vi "Maya2000 - set N coadd and integr time.vi"(4 "Intgration time\n[us]":u32=44444, 6 "numberOfScans\nToAverage":u32=1 min=1 step=1, 8 "error in (no error)":errorcluster, 9 "Array index of UV\nspectrometers":T1, 10 "Maya2000 basic values":T2[](array[typedef]), 11 ".NET Refnum in":refnum<k24>) -> (0 "error out":errorcluster, 1 "This instruments index":i32, 2 "This Maya´\nbasic info":T2, 3 ".NET Refnum out":refnum<k24>)   [LabVIEW 2015]
uses:
  Maya2000 Typedefs/Maya2000 basic info.ctl
  C:/Program Files (x86)/Ocean Optics/OmniDriver/OOI_HOME/NETOmniDriver-NET40.dll
  Maya2000 Typedefs/Basic info-array index of UV spectometers.ctl
  <vilib>/GPower/Error/Library/ErrorType.vi
  <vilib>/GPower/Error/Library/SplitAppended.vi
  <vilib>/GPower/Error/Library/SubVIs/ExplanationToError.vi
  <vilib>/dlg_ctls.llb/Space Constant.vi
  <vilib>/Utility/error.llb/Error Cluster From Error Code.vi
  <vilib>/Utility/error.llb/Trim Whitespace.vi
  <vilib>/Utility/error.llb/Error Code Database.vi
  <vilib>/GPower/Error/Library/SubVIs/SetStatus.vi
  <vilib>/GPower/Error/Library/AppendErrors.vi
  <vilib>/GPower/Error/Library/Append/AppendSingle.vi
  <vilib>/ErrorRing/Error Ring.xnode
  <vilib>/GPower/Error/GPError.lvlib
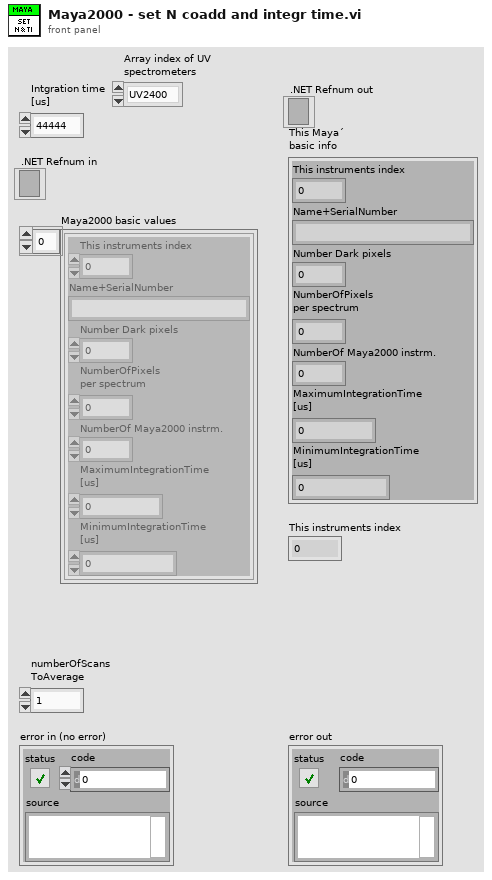
[diagram p1: front panel]
types:
  T1 = typedef "Basic info-array index of UV spectometers.ctl" = enum32{"UV2400", "UV600"}
  T2 = typedef "Maya2000 basic info.ctl" = cluster{"This instruments index":i32, "Name+SerialNumber":string, "Number Dark pixels":i32, "NumberOfPixels\nper spectrum":i32, "NumberOf Maya2000 instrm.":i32, "MaximumIntegrationTime\n[us]":i32, "MinimumIntegrationTime\n[us]":i32}
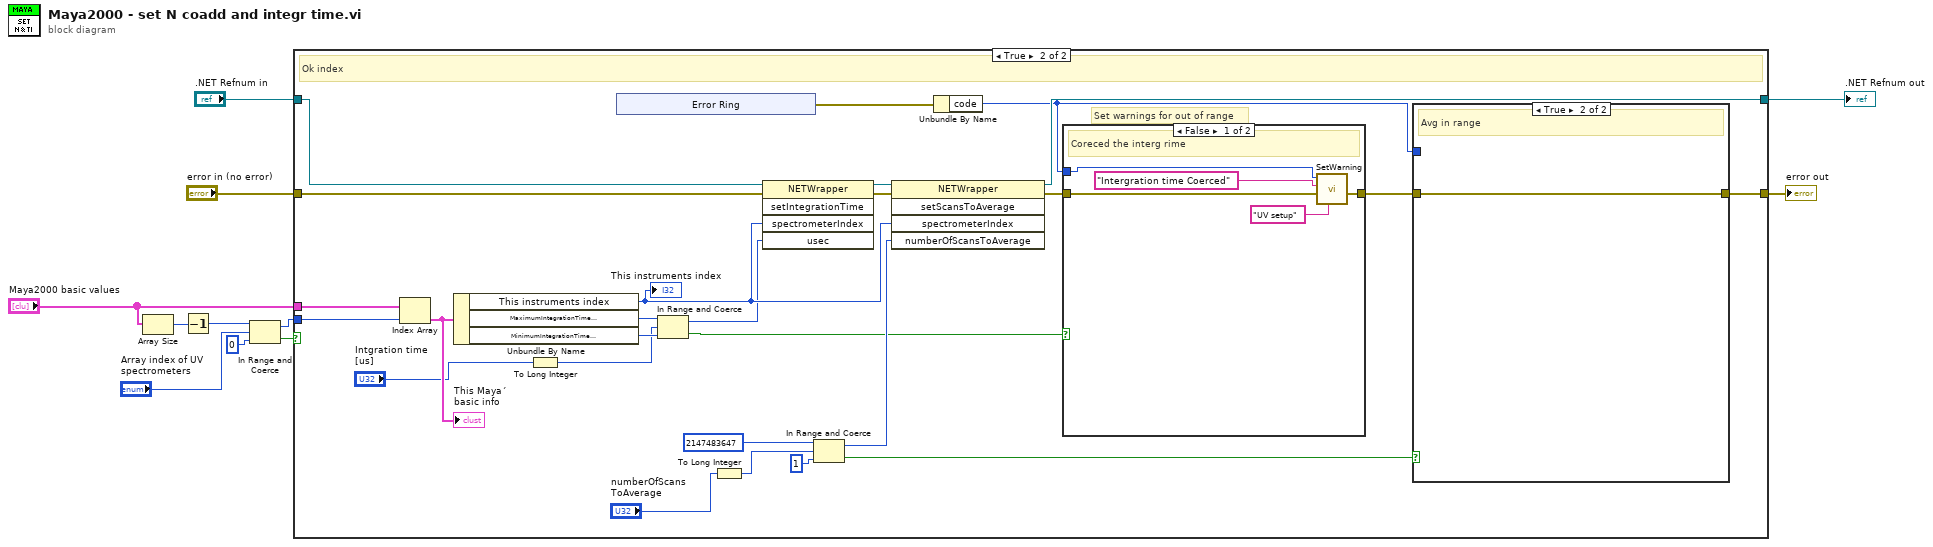
[diagram p0: block diagram]
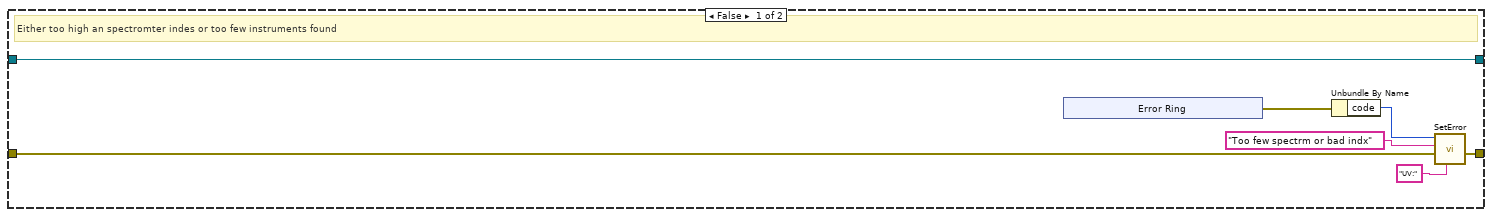
[diagram p2: hidden frame]
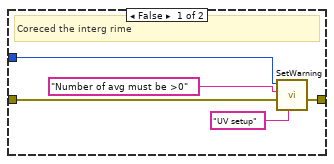
[diagram p3: hidden frame]
diagram:
  n1 = Array Size(array="Maya2000 basic values") -> (size(s)=w8:i32)
  n2 = Decrement(x=w8) -> (x-1=w9:i32)
  n3 = In Range and Coerce(upper limit=w9, x="Array index of UV\nspectrometers", lower limit=0) -> (coerced(x)=w10:u32, In Range?=w5:bool)
  n4 = case shown="True" w5 {
    tunnel: w10 -> [_ w48]
    tunnel: "Maya2000 basic values" -> [_ w47]
    tunnel: "error in (no error)" -> [w17 w40]
    tunnel: ".NET Refnum in" -> [w18 w39]
    tunnel: [w16 w29] -> w2
    tunnel: [w18 w38] -> w1
    frame False {
      # "Either too high an spectromter indes or too few instruments found"
      n5 = xnode "Error Ring"() -> ("error out"=w15:errorcluster)
      n6 = Unbundle By Name(w15) -> ("code"=w14:i32)
      n7 = call <vilib>:"SetError.vi"("Error label"="UV:", "Error in"=w17, "Error description"="Too few spectrm or bad indx", "Error code"=w14) -> ("Error out"=w16:errorcluster)  [unwired: 7 in]
    }
    frame True {
      # "Set warnings for out of range"
      # "Ok index"
      n8 = Index Array(array=w47, index=w48) -> (element=w44:T2)
      "This Maya´\nbasic info" <- w44
      n9 = Unbundle By Name(w44) -> ("This instruments index"=w24:i32, "MaximumIntegrationTime\n[us]"=w45:i32, "MinimumIntegrationTime\n[us]"=w46:i32)
      "This instruments index" <- w24
      n10 = To Long Integer(number="Intgration time\n[us]") -> (32bit integer=w28:i32)
      n11 = xnode "Error Ring"() -> ("error out"=w26:errorcluster)
      n12 = In Range and Coerce(upper limit=w45, x=w28, lower limit=w46) -> (coerced(x)=w23:i32, In Range?=w33:bool)
      n13 = To Long Integer(number="numberOfScans\nToAverage") -> (32bit integer=w27:i32)
      n14 = invoke class="NETWrapper" method="setIntegrationTime"(reference=w39, error in=w40, "spectrometerIndex"=w24, "usec"=w23) -> (reference out=w42:refnum<k24>, error out=w43:errorcluster)  [unwired: 1 in, 3 out]
      n15 = In Range and Coerce(upper limit=2147483647 ("lower limit"), x=w27, lower limit=1) -> (coerced(x)=w34:i32, In Range?=w30:bool)
      n16 = invoke class="NETWrapper" method="setScansToAverage"(reference=w42, error in=w43, "spectrometerIndex"=w24, "numberOfScansToAverage"=w34) -> (reference out=w38:refnum<k24>, error out=w32:errorcluster)  [unwired: 1 in, 3 out]
      n17 = Unbundle By Name(w26) -> ("code"=w25:i32)
      n18 = case shown="False" w33 {
        tunnel: w32 -> [w63 w64]
        tunnel: [w62 w64] -> w31
        tunnel: w25 -> [w59 _]
        frame False {
          # "Coreced the interg rime"
          n19 = call <vilib>:"SetWarning.vi"("Warning label"="UV setup", "Error in"=w63, "Warning description"="Intergration time Coerced", "Warning code"=w59) -> ("Error out"=w62:errorcluster)  [unwired: 7 in]
        }
        frame True {
          # "Integr tome is in range"
        }
      }
      n20 = case shown="True" w30 {
        tunnel: w31 -> [w57 w58]
        tunnel: [w56 w58] -> w29
        tunnel: w25 -> [w53 _]
        frame False {
          # "Coreced the interg rime"
          n21 = call <vilib>:"SetWarning.vi"("Warning label"="UV setup", "Error in"=w57, "Warning description"="Number of avg must be >0", "Warning code"=w53) -> ("Error out"=w56:errorcluster)  [unwired: 7 in]
        }
        frame True {
          # "Avg in range"
        }
      }
    }
  }
  "error out" <- w2
  ".NET Refnum out" <- w1
